vi "Demo PID Control.vi"() -> ()   [LabVIEW 2024, in "Revidyne Generator.lvlib"]
uses:
  Revidyne Generator.lvlib
  <vilib>/addons/control/pid/pid.llb/PID (DBL).vi
  <vilib>/addons/control/pid/NI_PID_pid.lvlib
panel:
  in  "Stop":bool
  in  "VISA":refnum<visa-resource-name>
  in  "PID Gains":T1={"Proportional Gain (Kc)"=1.0, "Integral Time (Ti, min)"=0.01, "Derivative Time (Td, min)"=0.0} {"Derivative Time (Td, min)" format="%.3g"; "Integral Time (Ti, min)" format="%.3g"; "Proportional Gain (Kc)" format="%.3g"}
  in  "Setpoint":dbl(slide)=1.0 scale=0.0..200.0
  out "Gauge":dbl(knob) scale=0.0..255.0
  out "Generator Data":cluster{"Setpoint":dbl, "Value":dbl}(graph) caption="Waveform Chart - Dark"
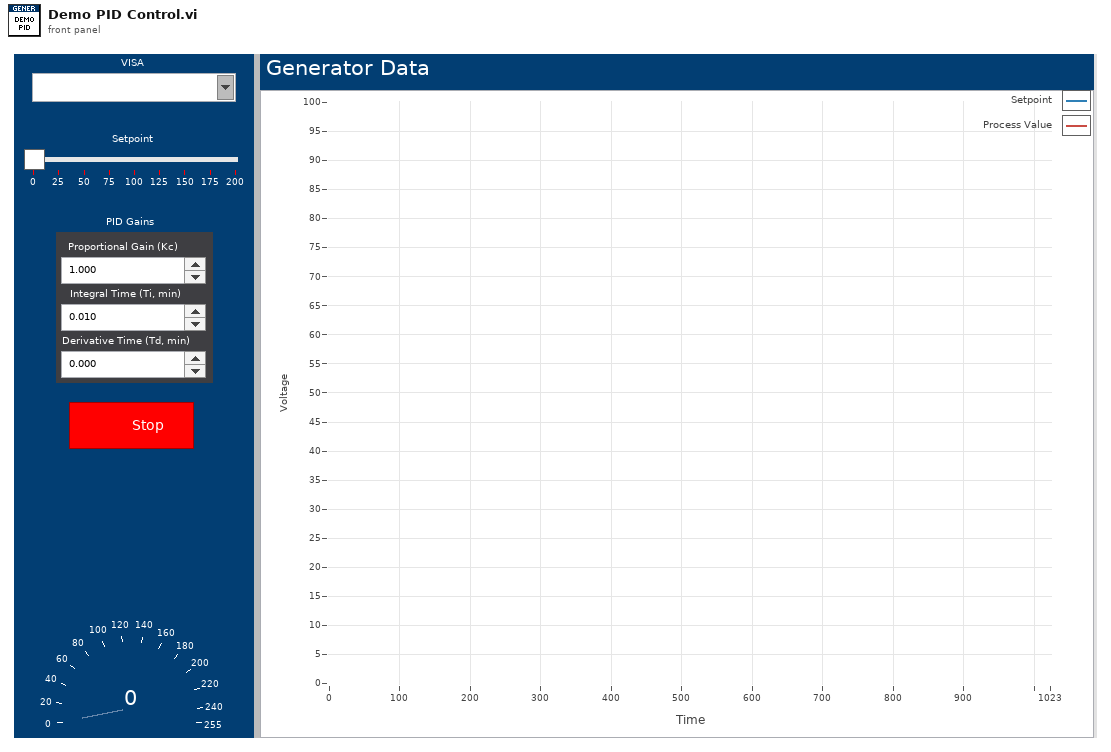
[diagram p1: front panel]
types:
  T1 = cluster{"Proportional Gain (Kc)":dbl, "Integral Time (Ti, min)":dbl, "Derivative Time (Td, min)":dbl}
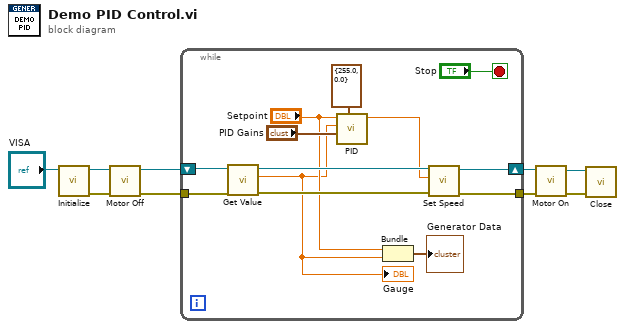
[diagram p0: block diagram]
diagram:
  n1 = call "Initialize.vi"("VISA resource name"="VISA") -> ("error out"=w9:errorcluster, "VISA resource name out"=w8:refnum<visa-resource-name>)  [unwired: 9 in]
  n2 = call "Motor Off.vi"("error in (no error)"=w9, "VISA resource name"=w8) -> ("error out"=w6:errorcluster, "VISA resource name out"=w7:refnum<visa-resource-name>)  [unwired: 8 in]
  n3 = while {
    shift-right: [w20] -> w3
    shift-left: w7 -> [w22]
    tunnel: w6 -> [w19]
    tunnel: [w17] -> w4
    stop <- "Stop" stop-if-true
    n4 = call "Get Value.vi"("error in (no error)"=w19, "VISA resource name"=w22) -> ("error out"=w18:errorcluster, "Value"=w10:dbl, "VISA resource name out"=w21:refnum<visa-resource-name>)  [unwired: 7 in]
    "Gauge" <- w10
    n5 = call-poly <vilib>:"PID.vi"("output range"=cluster{"output high":dbl, "output low":dbl} {"output high"=255.0, "output low"=0.0}, "PID gains"="PID Gains", "process variable"=w10, "setpoint"="Setpoint") -> ("output"=w16:dbl)  [unwired: 6 in, 1 out]
    n6 = Bundle("Setpoint"="Setpoint", "Value"=w10) -> (→"Generator Data":cluster{"Setpoint":dbl, "Value":dbl})  [unwired: 1 in]
    n7 = call "Set Speed.vi"("error in (no error)"=w18, "speed (0)"=w16, "VISA resource name"=w21) -> ("error out"=w17:errorcluster, "VISA resource name out"=w20:refnum<visa-resource-name>)  [unwired: 7 in]
  }
  n8 = call "Motor On.vi"("error in"=w4, "VISA resource name"=w3) -> ("error out"=w1:errorcluster, "VISA resource name out"=w2:refnum<visa-resource-name>)  [unwired: 8 in]
  n9 = call "Close.vi"("error in (no error)"=w1, "VISA resource name"=w2) -> ()  [unwired: 9 in, 1 out]
